vi "LVClass_CorrectionDataManager SetCommandMatrixPreferences.vi"(0 "CorrectionDataManager in":refnum<class "CorrectionDataManager.lvclass">, 7 "Prefs":T1, 11 "error in (no error)":errorcluster) -> (4 "CorrectionDataManager out":refnum<class "CorrectionDataManager.lvclass">, 15 "error out":errorcluster)   [LabVIEW 2020, in "CorrectionDataManager.lvclass"]
doc: "Command matrix computation preferences.\n\n<B>corrdata_managerIn</B> : CorrDataManager object.\n<B>corrdata_managerOut</B> : CorrDataManager object.\n<B>nb_kept_modes</B> : Number of influences (starting from the highest) to keep.\n<B>tilt_filtering</B> : If True, computed command matrix does not take tilt into account."
uses:
  CorrectionDataManager.lvclass
  InteractionMatrixToCommandMatrixParameters.ctl
  LVClass_CorrectionDataManager Read CorrectionDataManager.vi
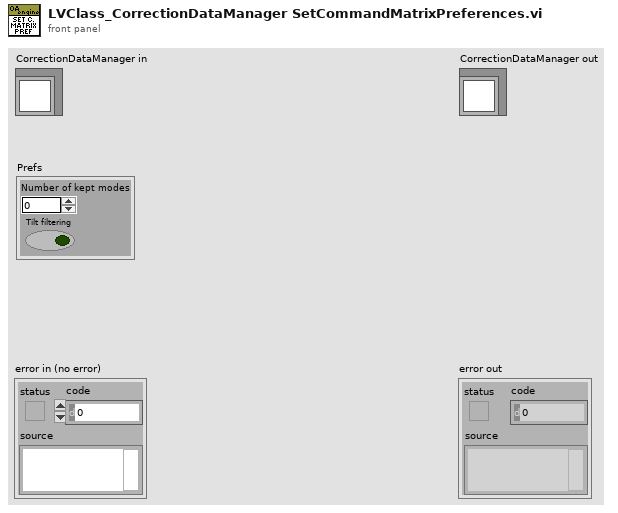
[diagram p1: front panel]
types:
  T1 = typedef "InteractionMatrixToCommandMatrixParameters.ctl" = cluster{"Number of kept modes":i32, "Tilt filtering":bool}
  T2 = typedef "ClassID.ctl" = i64
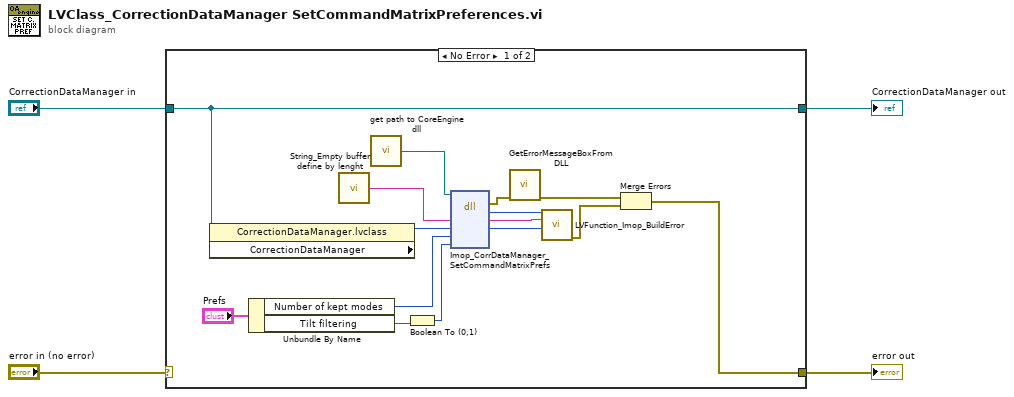
[diagram p0: block diagram]
diagram:
  n1 = case shown="No Error" "error in (no error)" {
    selector: "error in (no error)" -> [_ w21]
    tunnel: [w11 w21] -> w3
    tunnel: [w12 w20] -> w4
    tunnel: "CorrectionDataManager in" -> [w12 w20]
    frame No Error {
      n2 = property class="CorrectionDataManager.lvclass"(reference=w12) -> ("CorrectionDataManager"=w10:T2)  [unwired: 1 in, 2 out]
      n3 = Unbundle By Name("Prefs") -> ("Number of kept modes"=w8:i32, "Tilt filtering"=w7:bool)
      n4 = call "String_Empty buffer define by lenght.vi"() -> ("Empty buffer"=w17:string)  [unwired: 1 in]
      n5 = call "get path to CoreEngine dll.vi"() -> ("path to wavekit library"=w16:path)  [unwired: 14 in, 1 out]
      n6 = Boolean To (0,1)(Boolean=w7) -> (0, 1=w6:i16)
      n7 = dll-call lib="D:/soft/HASO_v3/SVN_trunk/ImOpCoreEngine4_LV2011/DLLs/c_interface_vc100.dll" fn="Imop_CorrDataManager_SetCommandMatrixPrefs"(path in=w16, "message"=w17, "WavefrontCorrection"=w10, "nb_kept_modes"=w8, "tilt_filtering"=w6) -> (error out=w15:errorcluster, "return type"=w19:i32, "message"=w18:string, "WavefrontCorrection"=w5:i64)  [unwired: 4 in, 1 out]
      n8 = call "GetErrorMessageBoxFromDLL.vi"("error IN"=w15) -> ("error OUT"=w14:errorcluster)  [unwired: 10 in]
      n9 = call "LVFunction_Imop_BuildError.vi"("code"=w19, "String to Prepend to source (\"\")"=w18, "Adresse"=w5) -> ("error out"=w13:errorcluster)  [unwired: 12 in]
      n10 = Merge Errors(w14, w13) -> (w11:errorcluster)
    }
    frame Error {
    }
  }
  "error out" <- w3
  "CorrectionDataManager out" <- w4
